vi "decode_request_from_serialport.vi"(6 "fast output index in":i32, 7 "fast output data in":dbl[][](array[numeric]), 8 "error in":errorcluster, 9 "FPGA VI Reference":refnum<k20>, 10 "request string":string, 11 "port name in":refnum<visa-resource-name>) -> (0 "error out":errorcluster, 2 "REQUEST_ID":u64, 3 "FPGA settings":T1={"Output settings"={"Relay Switch Matrix"=0, "Set output"=[0.0, 0.0, 0.0, 0.0], "set output?"=FALSE, "set relay matrix?"=FALSE}, "PID settings"={"PID input channel"=enum."PID Disabled", "PID output channel"=enum."PID Disabled", "PID gains"={"proportional gain"=0.0, "integral gain"=0.0, "derivative gain"=0.0, "filter coefficient"=0.0}, "PID output ranges"={"output high (Inf)"=0.0, "output low (-Inf)"=0.0}, "Setpoint for PID input chn"=0.0, "config PID gain?"=FALSE, "reset PID?"=FALSE, "config PID range?"=FALSE, "config PID input?"=FALSE, "config PID output?"=FALSE, "config PID setpoint?"=FALSE, "PID input scale factor"=1.0, "PID input offset"=0.0}, "NI9219 Settings"={"9219 Conversion Time"=enum."High Speed", "Input voltage range"=[0, 0, 0, 0], "config 9219 conversion time?"=FALSE, "config 9219 input range?"=FALSE}, "REQUEST_ID"=0, "requests"={"request_data"=FALSE, "request_system_status"=FALSE, "request_error_log"=FALSE}} {"REQUEST_ID" format="%x"; "NI9219 Settings"."Input voltage range" items=["+/- 60V", "+/- 15V", "+/- 4V", "+/- 1V", "+/- 125mV"]}, 4 "fast output index out":i32, 5 "fast output data out":dbl[][](array[numeric]))   [LabVIEW 2018]
uses:
  Type Def Ctrls/RT ctrls/FPGA parameter cluster.ctl
  Type Def Ctrls/FPGA ctrls/NI9219VoltageRange.ctl
  Type Def Ctrls/keywords for serial communication.ctl
  <vilib>/Utility/miscctls.llb/LVDateTimeRec.ctl
  <vilib>/FPGAPlugInAG/Dynamic/niLvFpga_Abort_Dynamic.vi
  <vilib>/FPGAPlugInAG/Dynamic/niLvFpga_Reset_Dynamic.vi
  <vilib>/FPGAPlugInAG/cRIO-9074/niLvFpga_Open_cRIO-9074.vi
  <vilib>/rvi/interface/common/dynamic/niFpgaDynamicAddResources.vi
  <vilib>/Utility/error.llb/Error Cluster From Error Code.vi
  <vilib>/rvi/errors/niLvFpgaAdjustHostInterfaceError.vi
  <vilib>/FPGAPlugInAG/Dynamic/niLvFpga_Close_Dynamic.vi
  <vilib>/nisyscfg/Close (System).vi
  <vilib>/rvi/interface/nirviMethod/nirviMethod.xnode
  <vilib>/rvi/interface/nirviOpenFPGA/nirviOpenFPGA.xnode
  FPGA Bitfiles/remotecontroller_FPGATarget_FPGAMain_RhGo+c1SRDI.lvbitx
  FPGA Main.vi
  <vilib>/rvi/interface/nirviReadWriteControl/nirviReadWriteControl.xnode
  <vilib>/rvi/interface/nirviCloseFPGA/nirviCloseFPGA.xnode
  <vilib>/nisyscfg/nisyscfg.lvlib
  NiFpgaLv.dll
  <vilib>/rvi/interface/Simulation/niFpgaSimulationCallBeginRW.vi
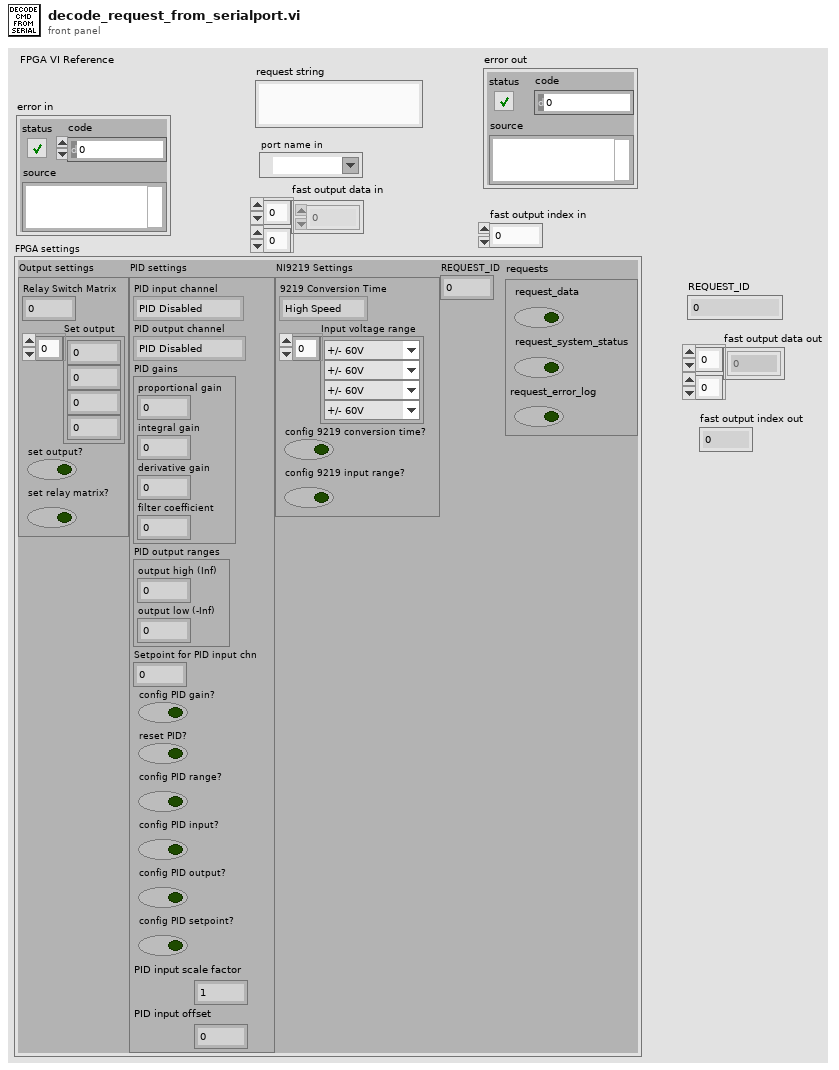
[diagram p1: front panel]
types:
  T1 = typedef "FPGA parameter cluster.ctl" = cluster{"Output settings":cluster{"Relay Switch Matrix":u32, "Set output":sgl[], "set output?":bool, "set relay matrix?":bool}, "PID settings":cluster{"PID input channel":enum16{"Output Channel 0", "Output Channel 1", "Output Channel 2", "Output Channel 3", "PID Disabled"}, "PID output channel":enum16{"Output Channel 0", "Output Channel 1", "Output Channel 2", "Output Channel 3", "PID Disabled"}, "PID gains":cluster{"proportional gain":sgl, "integral gain":sgl, "derivative gain":sgl, "filter coefficient":sgl}, "PID output ranges":cluster{"output high (Inf)":sgl, "output low (-Inf)":sgl}, "Setpoint for PID input chn":sgl, "config PID gain?":bool, "reset PID?":bool, "config PID range?":bool, "config PID input?":bool, "config PID output?":bool, "config PID setpoint?":bool, "PID input scale factor":sgl, "PID input offset":sgl}, "NI9219 Settings":cluster{"9219 Conversion Time":enum8{"High Speed", "Best 60 Hz Rejection", "Best 50 Hz Rejection", "High Resolution"}, "Input voltage range":T2[], "config 9219 conversion time?":bool, "config 9219 input range?":bool}, "REQUEST_ID":u64, "requests":cluster{"request_data":bool, "request_system_status":bool, "request_error_log":bool}}
  T2 = typedef "NI9219VoltageRange.ctl" = u8
  T3 = typedef "keywords for serial communication.ctl" = string[]
  T4 = enum16{"Safe State", "I/O with PID Control", "Fast Output Only", "NOT_READY"}
  T5 = typedef "LVDateTimeRec.ctl" = cluster{"fractional second":dbl, "second":i32, "minute":i32, "hour":i32, "day of month":i32, "month":i32, "year":i32, "day of week":i32, "day of year":i32, "DST":i32}
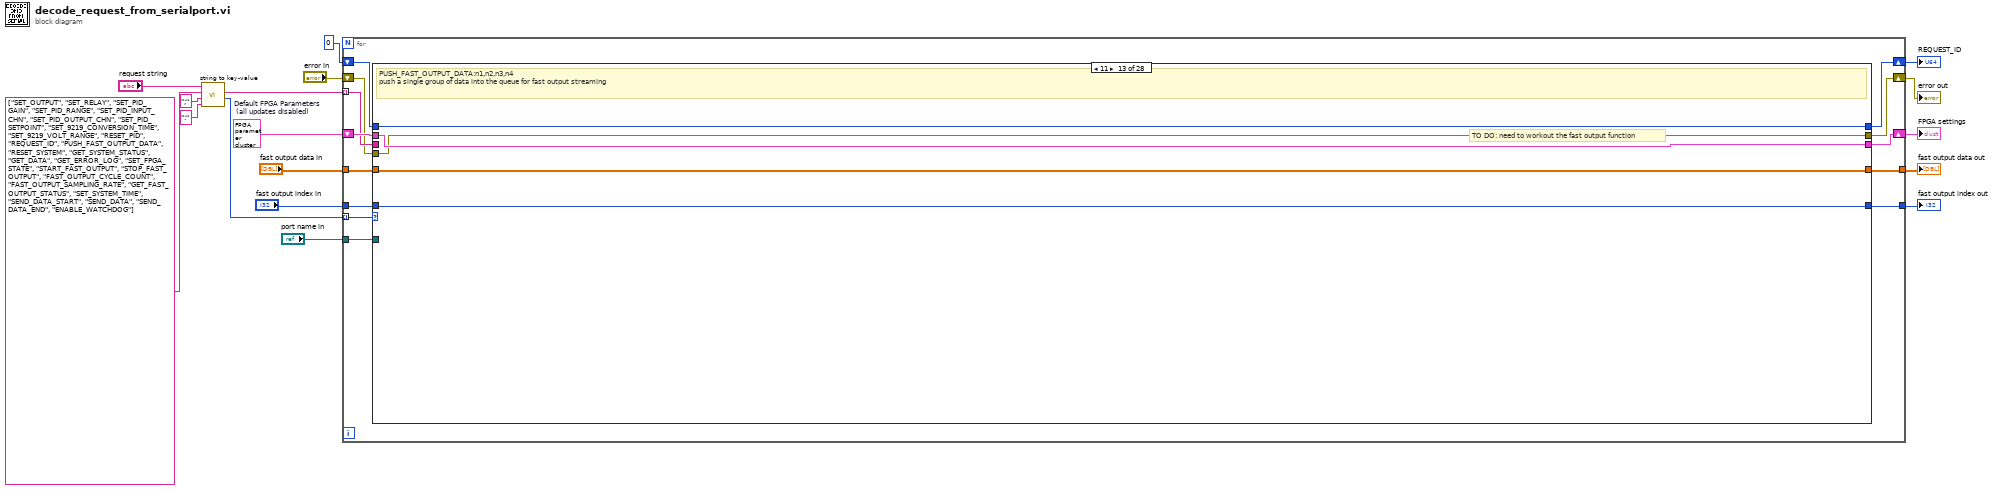
[diagram p0: block diagram]
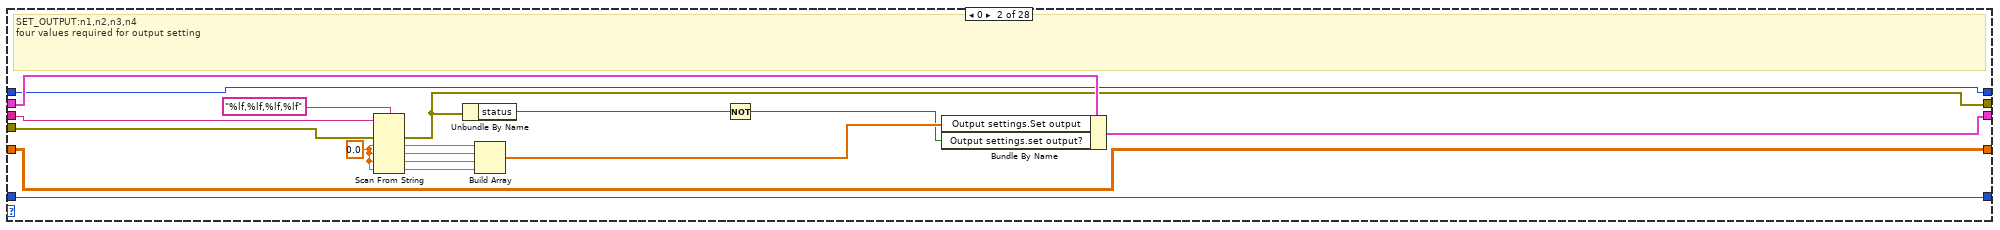
[diagram p3: hidden frame]
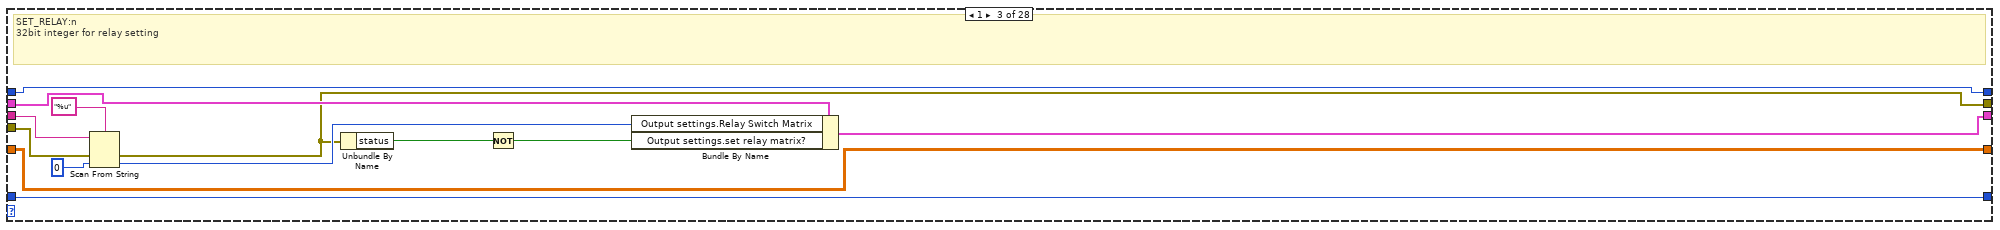
[diagram p4: hidden frame]
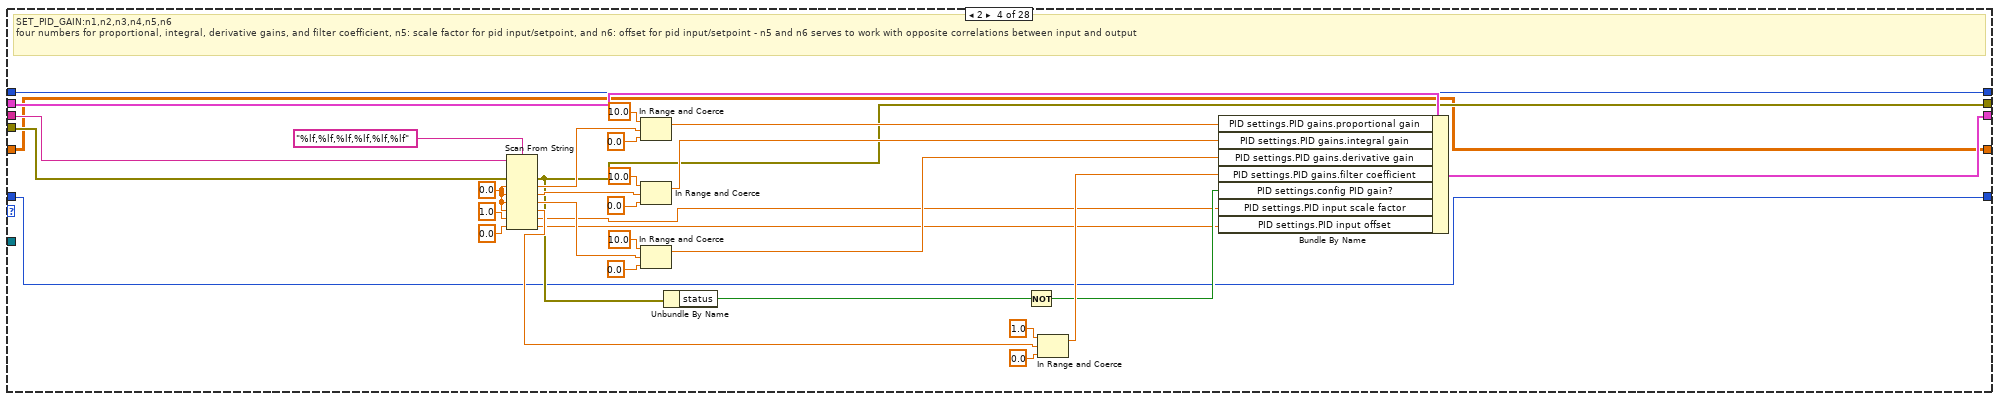
[diagram p5: hidden frame]
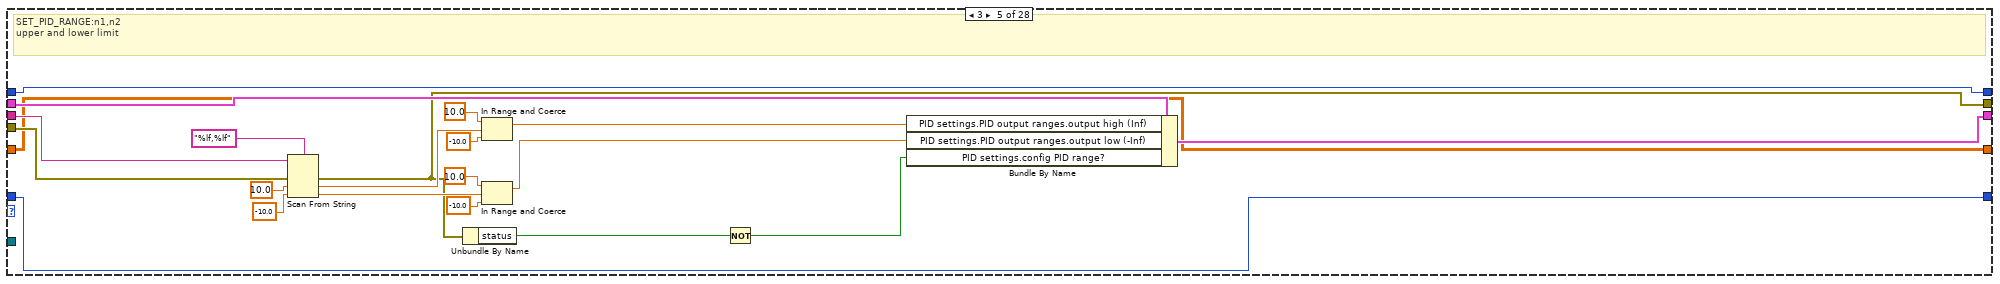
[diagram p6: hidden frame]
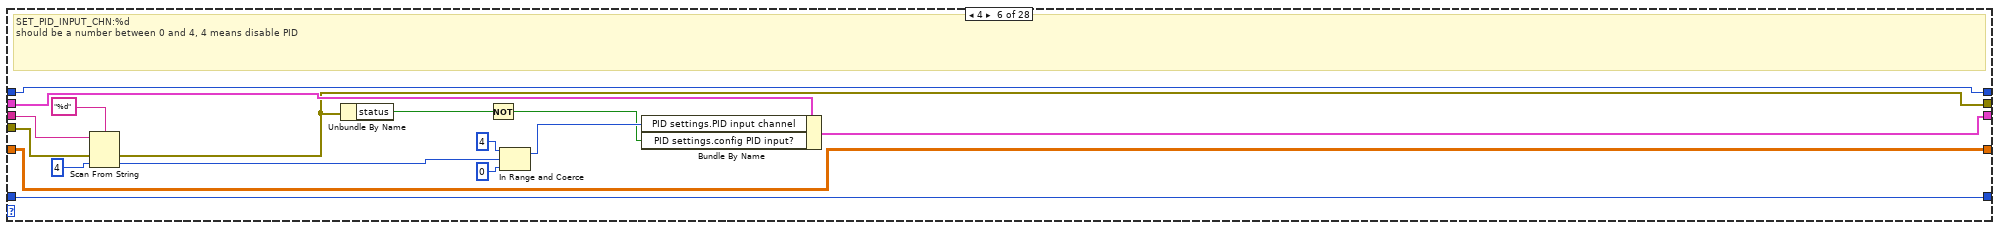
[diagram p7: hidden frame]
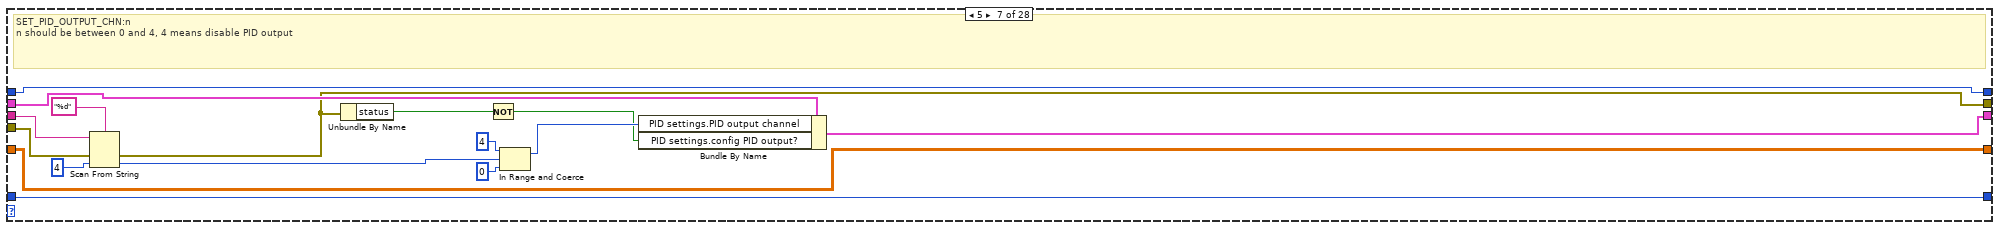
[diagram p8: hidden frame]
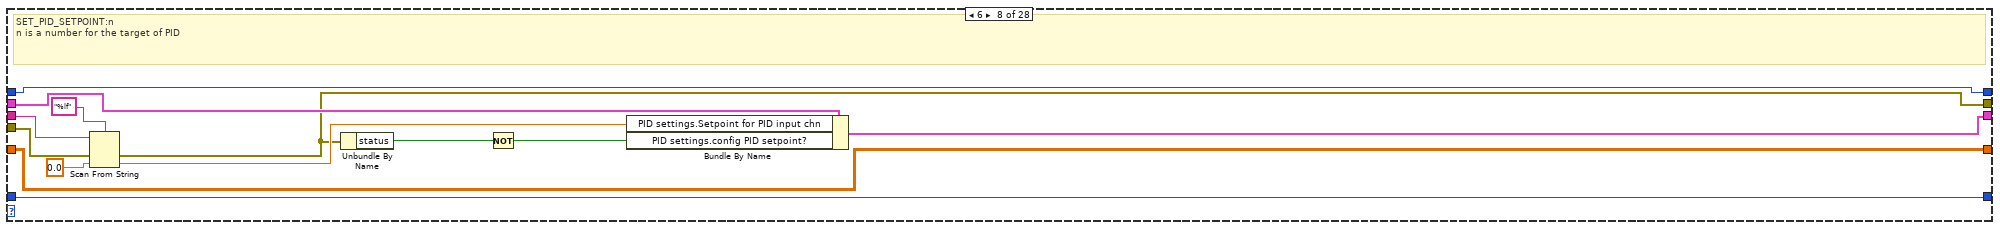
[diagram p9: hidden frame]
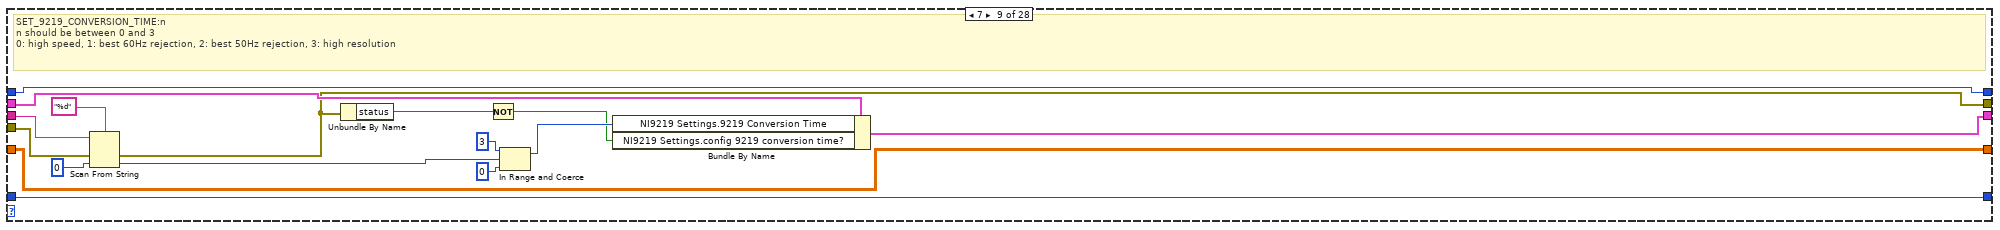
[diagram p10: hidden frame]
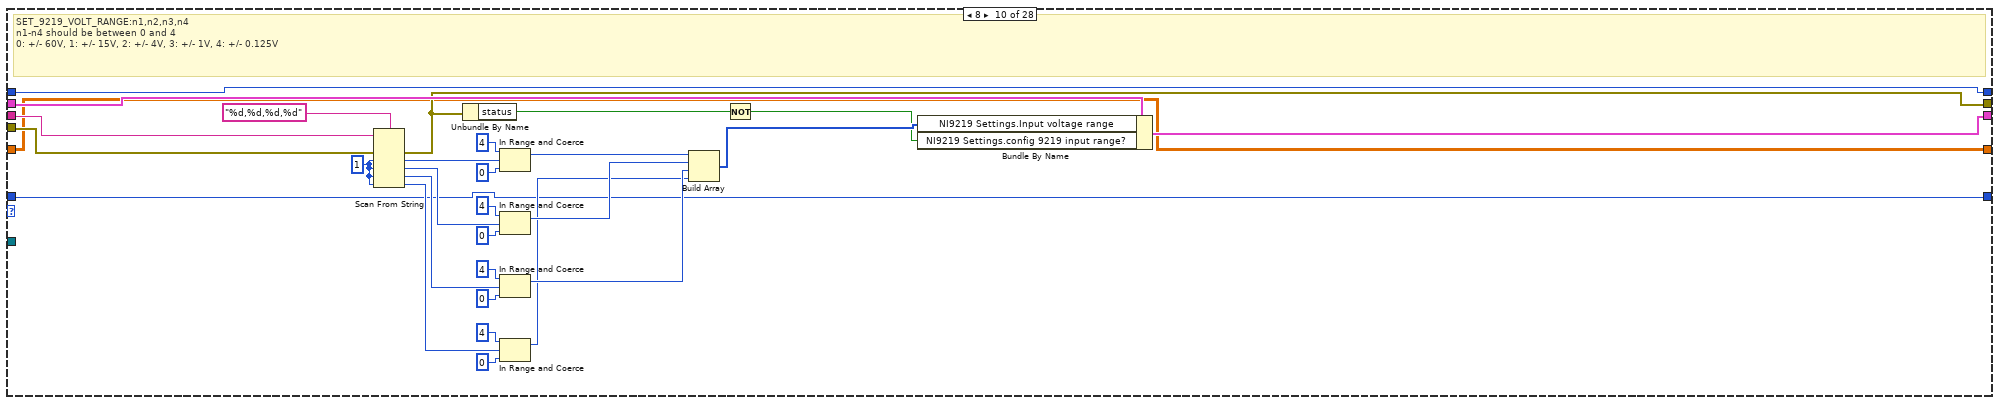
[diagram p11: hidden frame]
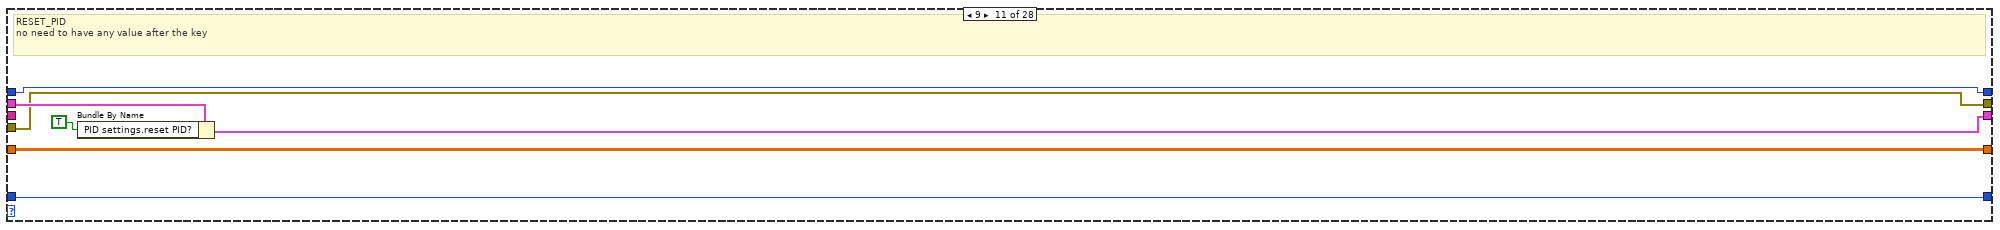
[diagram p12: hidden frame]
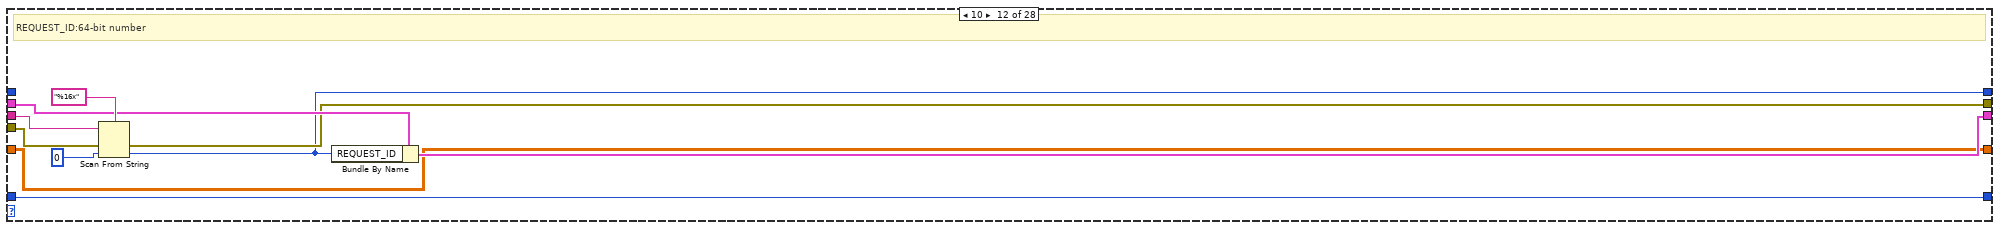
[diagram p13: hidden frame]
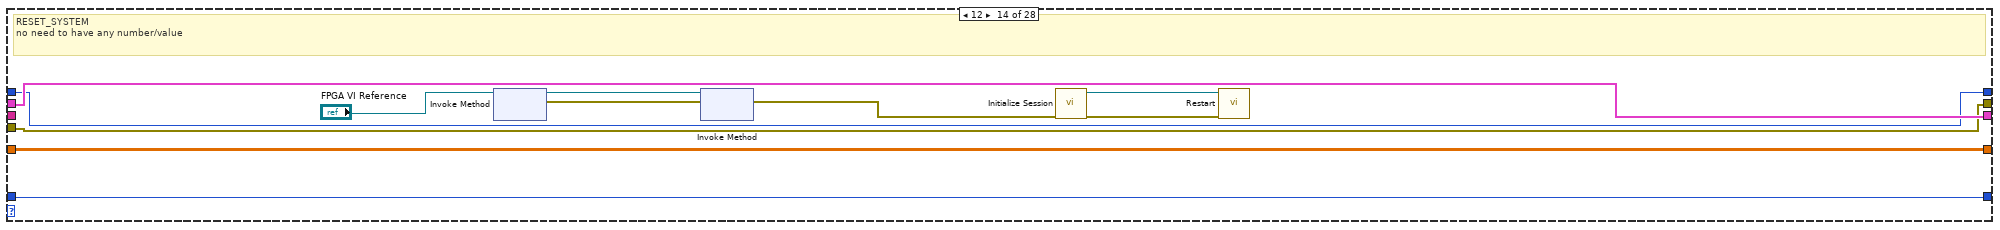
[diagram p14: hidden frame]
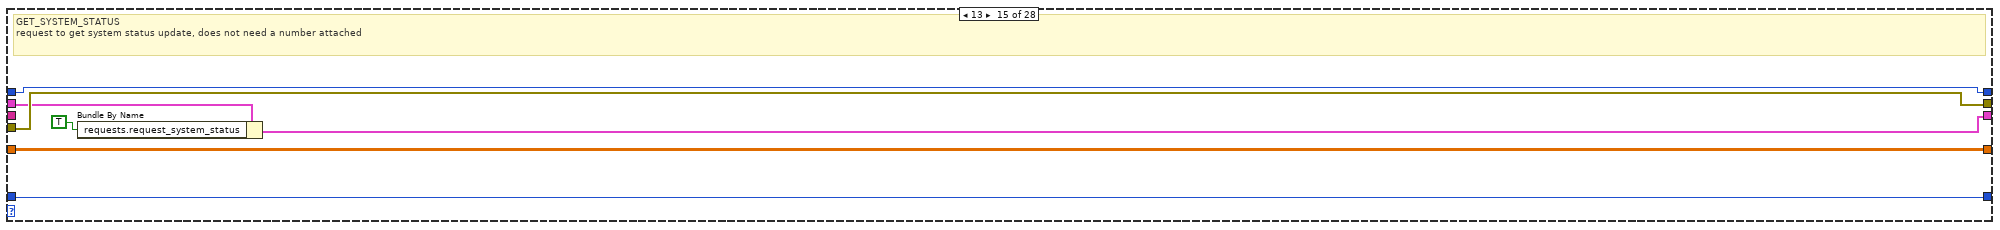
[diagram p15: hidden frame]
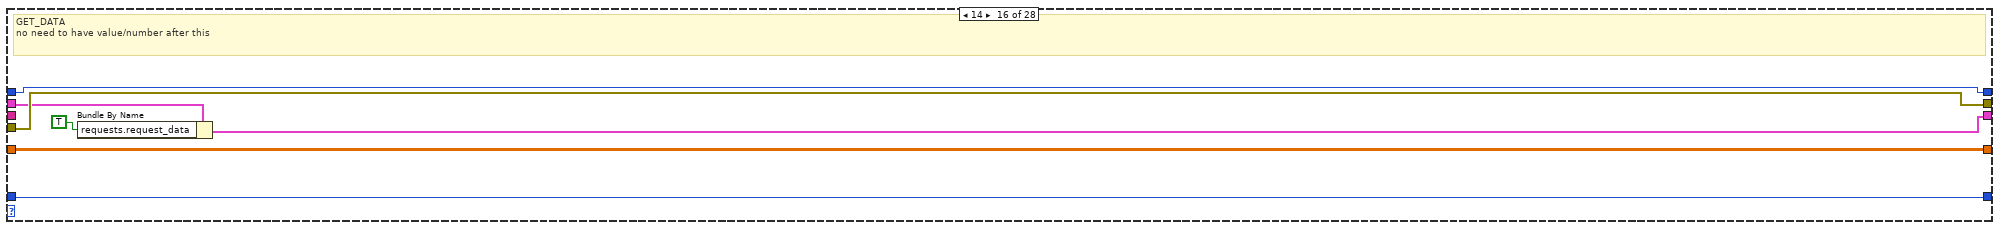
[diagram p16: hidden frame]
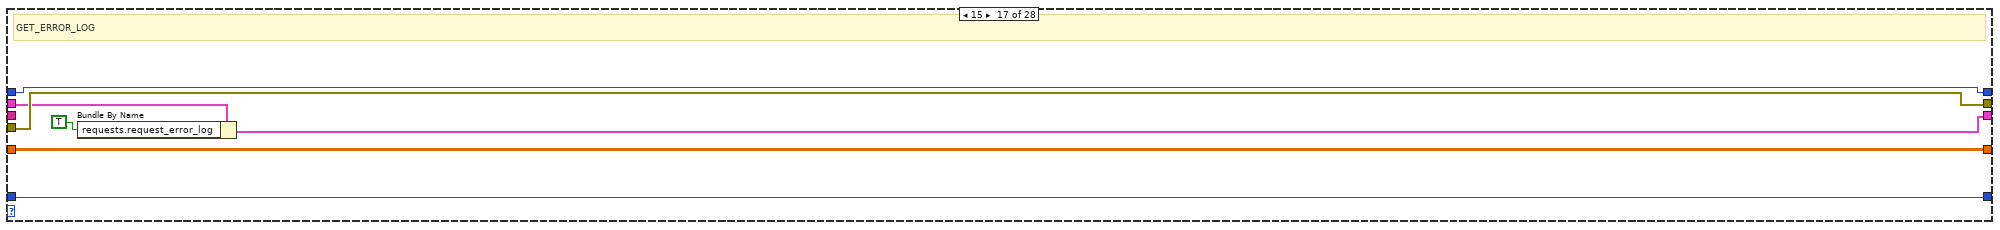
[diagram p17: hidden frame]
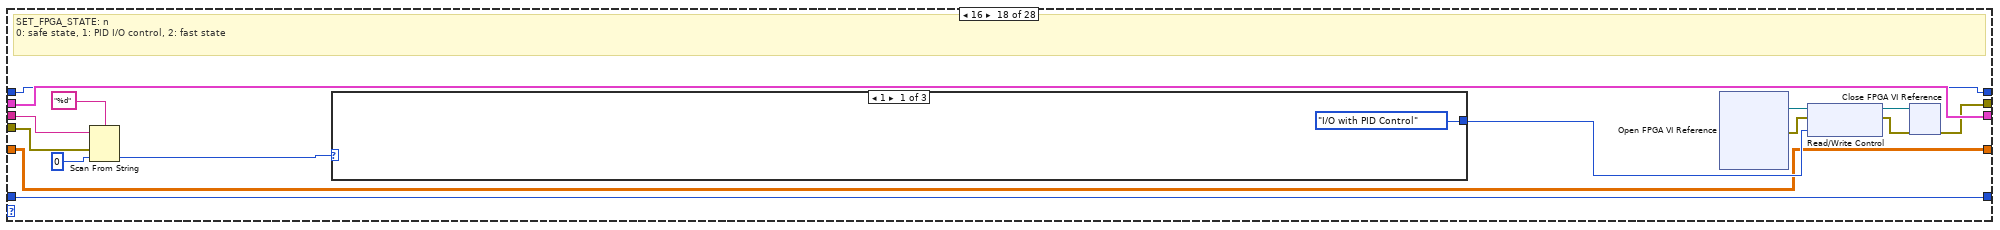
[diagram p18: hidden frame]
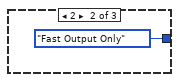
[diagram p19: hidden frame]
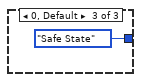
[diagram p20: hidden frame]
diagram:
  w15 = T1 {"Output settings"={"Relay Switch Matrix"=0, "Set output"=[0.0, 0.0, 0.0, 0.0], "set output?"=FALSE, "set relay matrix?"=FALSE}, "PID settings"={"PID input channel"=enum."PID Disabled", "PID output channel"=enum."PID Disabled", "PID gains"={"proportional gain"=0.0, "integral gain"=0.0, "derivative gain"=0.0, "filter coefficient"=0.0}, "PID output ranges"={"output high (Inf)"=0.0, "output low (-Inf)"=0.0}, "Setpoint for PID input chn"=0.0, "config PID gain?"=FALSE, "reset PID?"=FALSE, "config PID range?"=FALSE, "config PID input?"=FALSE, "config PID output?"=FALSE, "config PID setpoint?"=FALSE, "PID input scale factor"=1.0, "PID input offset"=0.0}, "NI9219 Settings"={"9219 Conversion Time"=enum."High Speed", "Input voltage range"=[1, 1, 1, 4], "config 9219 conversion time?"=FALSE, "config 9219 input range?"=FALSE}, "REQUEST_ID"=0, "requests"={"request_data"=FALSE, "request_system_status"=FALSE, "request_error_log"=FALSE}}  # Default FPGA Parameters  (all updates disabled)
  n1 = call "string to key-value.vi"("separation between key and value"=":", "separation between K-V sections"=";", "known key list"=T3 ["SET_OUTPUT", "SET_RELAY", "SET_PID_GAIN", "SET_PID_RANGE", "SET_PID_INPUT_CHN", "SET_PID_OUTPUT_CHN", "SET_PID_SETPOINT", "SET_9219_CONVERSION_TIME", "SET_9219_VOLT_RANGE", "RESET_PID", "REQUEST_ID", "PUSH_FAST_OUTPUT_DATA", "RESET_SYSTEM", "GET_SYSTEM_STATUS", "GET_DATA", "GET_ERROR_LOG", "SET_FPGA_STATE", "START_FAST_OUTPUT", "STOP_FAST_OUTPUT", "FAST_OUTPUT_CYCLE_COUNT", "FAST_OUTPUT_SAMPLING_RATE", "GET_FAST_OUTPUT_STATUS", "SET_SYSTEM_TIME", "SEND_DATA_START", "SEND_DATA", "SEND_DATA_END", "ENABLE_WATCHDOG"] ("key groups"), "input string"="request string") -> ("key index list"=w11:i32[], "value list"=w10:string[])  [unwired: 1 in, 1 out]
  n2 = for {
    shift-right: [w29] -> w16
    shift-left: w15 -> [w30]
    tunnel: w11 -> [w28] mode=indexing
    tunnel: w10 -> [w27] mode=indexing
    shift-right: [w25] -> w17
    shift-left: "error in" -> [w26]
    tunnel: "port name in" -> [w24]
    tunnel: [w23] -> w4
    tunnel: "fast output data in" -> [w22]
    tunnel: "fast output index in" -> [w21]
    tunnel: [w20] -> w3
    shift-right: [w19] -> w1
    shift-left: u64 0 ("default value 1") -> [w18]
    n3 = case shown="11" w28 {
      tunnel: w30 -> [w35 w52 w65 w97 w108 w128 w147 w160 w173 w193 w215 w222 w230 w241 w247 w254 w261 w269 w285 w290 w295 w300 w305 w311 w358 w370 w407 w414]
      tunnel: [w35 w51 w64 w77 w105 w126 w142 w158 w171 w187 w214 w221 w230 w241 w245 w253 w260 w269 w285 w290 w295 w300 w305 w311 w358 w370 w407 w414] -> w29
      tunnel: w27 -> [_ w50 w63 w96 w118 w134 w150 w163 w179 w208 _ w225 _ _ _ _ _ w273 _ _ _ _ _ w345 w356 w360 _ w418]
      tunnel: w26 -> [w34 w42 w58 w75 w104 w124 w141 w157 w170 w185 w212 w220 w229 w240 w248 w255 w262 w272 w284 w289 w294 w299 w304 w310 w355 w369 w406 w417]
      tunnel: [w34 w39 w56 w73 w102 w122 w138 w154 w167 w183 w212 w219 w229 w240 w248 w255 w262 w264 w284 w289 w294 w299 w304 w309 w354 w369 w406 w413] -> w25
      tunnel: w24 -> [_ _ _ _ _ _ _ _ _ _ _ _ _ _ _ _ _ _ _ _ _ _ _ _ _ _ _ _]
      tunnel: [w33 w38 w55 w72 w100 w121 w137 w153 w166 w182 w211 w218 w228 w233 w244 w251 w258 w268 w283 w288 w293 w298 w303 w308 w350 w367 w405 w412] -> w23
      tunnel: w22 -> [w33 w38 w55 w72 w100 w121 w137 w153 w166 w182 w211 w218 w228 w233 w244 w251 w258 w268 w283 w288 w293 w298 w303 w308 _ w366 w405 w412]
      tunnel: w21 -> [w32 w37 w54 w71 w99 w120 w136 w152 w165 w181 w210 w217 w227 w232 w243 w250 w257 w267 w282 w287 w292 w297 w302 w307 _ w365 _ w411]
      tunnel: [w32 w37 w54 w71 w99 w120 w136 w152 w165 w181 w210 w217 w227 w232 w243 w250 w257 w267 w282 w287 w292 w297 w302 w307 w349 w368 w402 w411] -> w20
      tunnel: [w31 w36 w53 w66 w98 w119 w135 w151 w164 w180 w209 w216 w226 w231 w242 w249 w256 w263 w281 w286 w291 w296 w301 w306 w346 w359 w401 w408] -> w19
      tunnel: w18 -> [w31 w36 w53 w66 w98 w119 w135 w151 w164 w180 w209 _ w226 w231 w242 w249 w256 w263 w281 w286 w291 w296 w301 w306 w346 w359 w401 w408]
      frame -1, Default {
      }
      frame 0 {
        w48 = 0.0 ("default value 1")
        # "SET_OUTPUT:n1,n2,n3,n4\nfour values required for output setting"
        n4 = Scan From String(format string="%lf,%lf,%lf,%lf", input string=w50, error in=w42, default 1=w48, default 2=w48, default 3=w48, default 4=w48) -> (error out=w39:errorcluster, output 1=w47:dbl, output 2=w46:dbl, output 3=w45:dbl, output 4=w44:dbl)  [unwired: 1 in, 2 out]
        n5 = Unbundle By Name(w39) -> ("status"=w41:bool)
        n6 = Build Array(w47, w46, w45, w44) -> (w43:dbl[])
        n7 = Not(x=w41) -> (.not. x?=w40:bool)
        n8 = Bundle By Name(cluster=w52, "Output settings.Set output"=w43, "Output settings.set output?"=w40) -> (w51:T1)
      }
      frame 1 {
        # "SET_RELAY:n\n32bit integer for relay setting"
        n9 = Scan From String(format string="%u", input string=w63, error in=w58, default 1=u32 0 ("default value 1")) -> (error out=w56:errorcluster, output 1=w60:u32)  [unwired: 1 in, 2 out]
        n10 = Unbundle By Name(w56) -> ("status"=w59:bool)
        n11 = Not(x=w59) -> (.not. x?=w57:bool)
        n12 = Bundle By Name(cluster=w65, "Output settings.Relay Switch Matrix"=w60, "Output settings.set relay matrix?"=w57) -> (w64:T1)
      }
      frame 2 {
        w94 = 0.0 ("default value 4")
        # "SET_PID_GAIN:n1,n2,n3,n4,n5,n6\nfour numbers for proportional, integral, derivative gains, and filter coefficient, n5: scale factor for pid input/setpoint, and n6: offset for pid input/setpoint - n5 and n6 serves to work with opposite correlations between input and output"
        n13 = Scan From String(format string="%lf,%lf,%lf,%lf,%lf,%lf", input string=w96, error in=w75, default 1=w94, default 2=w94, default 3=w94, default 4=w94, default 5=1.0 ("default value 5"), default 6=0.0 ("default value 6")) -> (error out=w73:errorcluster, output 1=w93:dbl, output 2=w83:dbl, output 3=w81:dbl, output 4=w78:dbl, output 5=w68:dbl, output 6=w67:dbl)  [unwired: 1 in, 2 out]
        n14 = In Range and Coerce(upper limit=10.0, x=w93, lower limit=0.0) -> (coerced(x)=w90:dbl)  [unwired: 1 out]
        n15 = In Range and Coerce(upper limit=10.0, x=w83, lower limit=0.0) -> (coerced(x)=w82:dbl)  [unwired: 1 out]
        n16 = In Range and Coerce(upper limit=10.0, x=w81, lower limit=0.0) -> (coerced(x)=w80:dbl)  [unwired: 1 out]
        n17 = Unbundle By Name(w73) -> ("status"=w76:bool)
        n18 = Not(x=w76) -> (.not. x?=w74:bool)
        n19 = In Range and Coerce(upper limit=1.0, x=w78, lower limit=0.0) -> (coerced(x)=w79:dbl)  [unwired: 1 out]
        n20 = Bundle By Name(cluster=w97, "PID settings.PID gains.proportional gain"=w90, "PID settings.PID gains.integral gain"=w82, "PID settings.PID gains.derivative gain"=w80, "PID settings.PID gains.filter coefficient"=w79, "PID settings.config PID gain?"=w74, "PID settings.PID input scale factor"=w68, "PID settings.PID input offset"=w67) -> (w77:T1)
      }
      frame 3 {
        # "SET_PID_RANGE:n1,n2\nupper and lower limit"
        n21 = Scan From String(format string="%lf,%lf", input string=w118, error in=w104, default 1=10.0 ("default value 1"), default 2=-10.0 ("default value 2")) -> (error out=w102:errorcluster, output 1=w114:dbl, output 2=w109:dbl)  [unwired: 1 in, 2 out]
        n22 = Unbundle By Name(w102) -> ("status"=w103:bool)
        n23 = In Range and Coerce(upper limit=10.0, x=w114, lower limit=-10.0) -> (coerced(x)=w107:dbl)  [unwired: 1 out]
        n24 = In Range and Coerce(upper limit=10.0, x=w109, lower limit=-10.0) -> (coerced(x)=w106:dbl)  [unwired: 1 out]
        n25 = Not(x=w103) -> (.not. x?=w101:bool)
        n26 = Bundle By Name(cluster=w108, "PID settings.PID output ranges.output high (Inf)"=w107, "PID settings.PID output ranges.output low (-Inf)"=w106, "PID settings.config PID range?"=w101) -> (w105:T1)
      }
      frame 4 {
        # "SET_PID_INPUT_CHN:%d\nshould be a number between 0 and 4, 4 means disable PID"
        n27 = Scan From String(format string="%d", input string=w134, error in=w124, default 1=4 ("default value 1")) -> (error out=w122:errorcluster, output 1=w131:i32)  [unwired: 1 in, 2 out]
        n28 = Unbundle By Name(w122) -> ("status"=w125:bool)
        n29 = Not(x=w125) -> (.not. x?=w123:bool)
        n30 = In Range and Coerce(upper limit=4, x=w131, lower limit=0) -> (coerced(x)=w127:i32)  [unwired: 1 out]
        n31 = Bundle By Name(cluster=w128, "PID settings.PID input channel"=w127, "PID settings.config PID input?"=w123) -> (w126:T1)
      }
      frame 5 {
        # "SET_PID_OUTPUT_CHN:n\nn should be between 0 and 4, 4 means disable PID output"
        n32 = Scan From String(format string="%d", input string=w150, error in=w141, default 1=4 ("default value 1")) -> (error out=w138:errorcluster, output 1=w146:i32)  [unwired: 1 in, 2 out]
        n33 = Unbundle By Name(w138) -> ("status"=w140:bool)
        n34 = Not(x=w140) -> (.not. x?=w139:bool)
        n35 = In Range and Coerce(upper limit=4, x=w146, lower limit=0) -> (coerced(x)=w143:i32)  [unwired: 1 out]
        n36 = Bundle By Name(cluster=w147, "PID settings.PID output channel"=w143, "PID settings.config PID output?"=w139) -> (w142:T1)
      }
      frame 6 {
        # "SET_PID_SETPOINT:n\nn is a number for the target of PID"
        n37 = Scan From String(format string="%lf", input string=w163, error in=w157, default 1=0.0 ("default value 1")) -> (error out=w154:errorcluster, output 1=w159:dbl)  [unwired: 1 in, 2 out]
        n38 = Unbundle By Name(w154) -> ("status"=w156:bool)
        n39 = Not(x=w156) -> (.not. x?=w155:bool)
        n40 = Bundle By Name(cluster=w160, "PID settings.Setpoint for PID input chn"=w159, "PID settings.config PID setpoint?"=w155) -> (w158:T1)
      }
      frame 7 {
        # "SET_9219_CONVERSION_TIME:n\nn should be between 0 and 3\n0: high speed, 1: best 60Hz rejection, 2: best 50Hz rejection, 3: high resolution"
        n41 = Scan From String(format string="%d", input string=w179, error in=w170, default 1=0 ("default value 1")) -> (error out=w167:errorcluster, output 1=w176:i32)  [unwired: 1 in, 2 out]
        n42 = Unbundle By Name(w167) -> ("status"=w169:bool)
        n43 = Not(x=w169) -> (.not. x?=w168:bool)
        n44 = In Range and Coerce(upper limit=3, x=w176, lower limit=0) -> (coerced(x)=w172:i32)  [unwired: 1 out]
        n45 = Bundle By Name(cluster=w173, "NI9219 Settings.9219 Conversion Time"=w172, "NI9219 Settings.config 9219 conversion time?"=w168) -> (w171:T1)
      }
      frame 8 {
        w206 = 1 ("default value 1")
        # "SET_9219_VOLT_RANGE:n1,n2,n3,n4\nn1-n4 should be between 0 and 4\n0: +/- 60V, 1: +/- 15V, 2: +/- 4V, 3: +/- 1V, 4: +/- 0.125V"
        n46 = Scan From String(format string="%d,%d,%d,%d", input string=w208, error in=w185, default 1=w206, default 2=w206, default 3=w206, default 4=w206) -> (error out=w183:errorcluster, output 1=w205:i32, output 2=w195:i32, output 3=w196:i32, output 4=w194:i32)  [unwired: 1 in, 2 out]
        n47 = Unbundle By Name(w183) -> ("status"=w186:bool)
        n48 = In Range and Coerce(upper limit=4, x=w205, lower limit=0) -> (coerced(x)=w192:i32)  [unwired: 1 out]
        n49 = In Range and Coerce(upper limit=4, x=w195, lower limit=0) -> (coerced(x)=w191:i32)  [unwired: 1 out]
        n50 = In Range and Coerce(upper limit=4, x=w196, lower limit=0) -> (coerced(x)=w190:i32)  [unwired: 1 out]
        n51 = In Range and Coerce(upper limit=4, x=w194, lower limit=0) -> (coerced(x)=w189:i32)  [unwired: 1 out]
        n52 = Build Array(w192, w191, w190, w189) -> (w188:i32[])
        n53 = Not(x=w186) -> (.not. x?=w184:bool)
        n54 = Bundle By Name(cluster=w193, "NI9219 Settings.Input voltage range"=w188, "NI9219 Settings.config 9219 input range?"=w184) -> (w187:T1)
      }
      frame 9 {
        # "RESET_PID\nno need to have any value after the key"
        n55 = Bundle By Name(cluster=w215, "PID settings.reset PID?"=TRUE) -> (w214:T1)
      }
      frame 10 {
        # "REQUEST_ID:64-bit number"
        n56 = Scan From String(format string="%16x", input string=w225, error in=w220, default 1=u64 0 ("default value 1")) -> (error out=w219:errorcluster, output 1=w216:u64)  [unwired: 1 in, 2 out]
        n57 = Bundle By Name(cluster=w222, "REQUEST_ID"=w216) -> (w221:T1)
      }
      frame 11 {
        # "TO DO: need to workout the fast output function"
        # "PUSH_FAST_OUTPUT_DATA:n1,n2,n3,n4\npush a single group of data into the queue for fast output streaming"
      }
      frame 12 {
        # "RESET_SYSTEM\nno need to have any number/value"
        n58 = xnode "Invoke Method"("FPGA VI Reference In"="FPGA VI Reference") -> ("FPGA VI Reference Out"=w235:refnum<k20>, "error out"=w236:errorcluster)  [unwired: 1 in]
        n59 = xnode "Invoke Method"("FPGA VI Reference In"=w235, "error in"=w236) -> ("error out"=w234:errorcluster)  [unwired: 1 out]
        n60 = call <vilib>:"Initialize Session.vi"("error in (no error)"=w234) -> ("error out"=w238:errorcluster, "Session out"=w239:refnum<k21>)  [unwired: 9 in]
        n61 = call <vilib>:"Restart.vi"("error in (no error)"=w238, "Session in"=w239) -> ()  [unwired: 7 in, 3 out]
      }
      frame 13 {
        # "GET_SYSTEM_STATUS\nrequest to get system status update, does not need a number attached"
        n62 = Bundle By Name(cluster=w247, "requests.request_system_status"=TRUE) -> (w245:T1)
      }
      frame 14 {
        # "GET_DATA\nno need to have value/number after this"
        n63 = Bundle By Name(cluster=w254, "requests.request_data"=TRUE) -> (w253:T1)
      }
      frame 15 {
        # "GET_ERROR_LOG"
        n64 = Bundle By Name(cluster=w261, "requests.request_error_log"=TRUE) -> (w260:T1)
      }
      frame 16 {
        # "SET_FPGA_STATE: n\n0: safe state, 1: PID I/O control, 2: fast state"
        n65 = Scan From String(format string="%d", input string=w273, error in=w272, default 1=0 ("default value 1")) -> (output 1=w271:i32)  [unwired: 1 in, 3 out]
        n66 = case shown="1" w271 {
          tunnel: [T4."I/O with PID Control" ("FPGA state") T4."Fast Output Only" ("FPGA state") T4."Safe State" ("FPGA state")] -> w270
          frame 1 {
          }
          frame 2 {
          }
          frame 0, Default {
          }
        }
        n67 = xnode "Open FPGA VI Reference"() -> ("FPGA VI Reference Out"=w277:refnum<k20>, "error out"=w276:errorcluster)  [unwired: 2 in]
        n68 = xnode "Read/Write Control"("FPGA VI Reference In"=w277, "error in"=w276, "FPGA state"=w270) -> ("FPGA VI Reference Out"=w266:refnum<k20>, "error out"=w265:errorcluster)
        n69 = xnode "Close FPGA VI Reference"("FPGA VI Reference In"=w266, "error in"=w265) -> ("error out"=w264:errorcluster)
      }
      frame 17 {
      }
      frame 18 {
      }
      frame 19 {
      }
      frame 20 {
      }
      frame 21 {
      }
      frame 22 {
        w343 = 0 ("default value 2")
        # "SET_SYSTEM_TIME:n1/n2/n3/n4/n5/n6\nn1: Month, n2: Day, n3: Year, n4: hour, n5: minute, n6: second, 24 hour format"
        n70 = Scan From String(format string="%d/%d/%d/%d/%d/%d", input string=w345, default 1=w343, default 2=w343, default 3=w343, default 4=w343, default 5=w343, default 6=w343) -> (output 1=w342:i32, output 2=w337:i32, output 3=w334:i32, output 4=w331:i32, output 5=w328:i32, output 6=w325:i32)  [unwired: 2 in, 3 out]
        n71 = In Range and Coerce(upper limit=12, x=w342, lower limit=1) -> (coerced(x)=w322:i32)  [unwired: 1 out]
        n72 = In Range and Coerce(upper limit=31, x=w337, lower limit=1) -> (coerced(x)=w320:i32)  [unwired: 1 out]
        n73 = In Range and Coerce(upper limit=23, x=w331, lower limit=0) -> (coerced(x)=w319:i32)  [unwired: 1 out]
        n74 = In Range and Coerce(upper limit=59, x=w328, lower limit=0) -> (coerced(x)=w318:i32)  [unwired: 1 out]
        n75 = In Range and Coerce(upper limit=59, x=w325, lower limit=0) -> (coerced(x)=w317:i32)  [unwired: 1 out]
        n76 = In Range and Coerce(upper limit=9999, x=w334, lower limit=0) -> (coerced(x)=w321:i32)  [unwired: 1 out]
        n77 = Bundle By Name(cluster=T5 {"fractional second"=0.0, "second"=0, "minute"=0, "hour"=0, "day of month"=0, "month"=0, "year"=0, "day of week"=0, "day of year"=0, "DST"=0} ("date time rec"), "year"=w321, "month"=w322, "day of month"=w320, "hour"=w319, "minute"=w318, "second"=w317) -> (w316:T5)
        n78 = Date/Time To Seconds(2:w316) -> (0:w324:timestamp)  [unwired: 1 in]
        n79 = call <vilib>:"Initialize Session.vi"("error in (no error)"=w310) -> ("error out"=w312:errorcluster, "Session out"=w315:refnum<k21>)  [unwired: 9 in]
        n80 = call <vilib>:"Set Time.vi"("error in (no error)"=w312, "Time"=w324, "Session in (localhost)"=w315) -> ("error out"=w314:errorcluster, "Session out"=w313:refnum<k21>)  [unwired: 5 in, 2 out]
        n81 = call-poly <vilib>:"Close.vi"("error in (no error)"=w314, "Session in"=w313) -> ("error out"=w309:errorcluster)  [unwired: 9 in]
      }
      frame 23 {
        w349 = 0 ("default value 1")
        # "SEND_DATA_START:n\nn is the total number of points"
        n82 = Scan From String(format string="%d", input string=w356, error in=w355, default 1=w349) -> (error out=w354:errorcluster, output 1=w352:i32)  [unwired: 1 in, 2 out]
        n83 = Greater Than 0?(x=w352) -> (x > 0?=w353:bool)
        n84 = Select(t=w352, s=w353, f=w349) -> (s? t:f=w347:i32)
        n85 = Initialize Array(0.0 ("element"), w347, 5 ("dimension size")) -> (w350:dbl[][])
      }
      frame 24 {
        # "SEND_DATA:n1,n2,n3,n4,n5\nn1,n2,n3,n4: voltage for output channels, n5: duration (counts of ticks, minimal 1)"
        n86 = Array Size(array=w366) -> (size(s)=w363:i32[])
        n87 = Index Array(array=w363, index=0) -> (element=w361:i32)
        n88 = Less?(x=w365, y=w361) -> (x < y?=w364:bool)
        n89 = case shown="True" w364 {
          tunnel: [w372 w398] -> w368
          tunnel: [w371 w397] -> w367
          tunnel: w366 -> [w371 w393]
          tunnel: w365 -> [w372 w381]
          tunnel: w360 -> [_ w373]
          frame False {
          }
          frame True {
            w392 = 1 ("default value 2")
            w374 = 0.0 ("default value 1")
            n90 = Increment(x=w381) -> (x+1=w398:i32)
            n91 = Scan From String(format string="%lf,%lf,%lf,%lf,%d", input string=w373, default 1=w374, default 2=w374, default 3=w374, default 4=w374, default 5=w392) -> (output 1=w396:dbl, output 2=w384:dbl, output 3=w383:dbl, output 4=w382:dbl, output 5=w385:i32)  [unwired: 2 in, 3 out]
            n92 = Greater Or Equal?(x=w385, y=w392) -> (x >= y?=w399:bool)
            n93 = In Range and Coerce(upper limit=10.0, x=w396, lower limit=-10.0) -> (coerced(x)=w380:dbl)  [unwired: 1 out]
            n94 = In Range and Coerce(upper limit=10.0, x=w384, lower limit=-10.0) -> (coerced(x)=w379:dbl)  [unwired: 1 out]
            n95 = In Range and Coerce(upper limit=10.0, x=w383, lower limit=-10.0) -> (coerced(x)=w378:dbl)  [unwired: 1 out]
            n96 = In Range and Coerce(upper limit=10.0, x=w382, lower limit=-10.0) -> (coerced(x)=w377:dbl)  [unwired: 1 out]
            n97 = Select(t=w385, s=w399, f=w392) -> (s? t:f=w376:i32)
            n98 = Build Array(w380, w379, w378, w377, w376) -> (w375:dbl[])
            n99 = Replace Array Subset(array=w393, new element=w375, index (row)=w381) -> (w397:dbl[][])  [unwired: 1 in]
          }
        }
      }
      frame 25 {
        # "SEND_DATA_END"
        n100 = Array Size(array=w405) -> (size(s)=w404:i32[])
        n101 = Index Array(array=w404, index=0) -> (element=w402:i32)
      }
      frame 26 {
        # "SWITCH_WATCHDOG"
        n102 = Scan From String(format string="%d", input string=w418, error in=w417, default 1=1 ("default value 1")) -> (error out=w413:errorcluster, output 1=w416:i32)  [unwired: 1 in, 2 out]
        n103 = xnode "Open FPGA VI Reference"() -> ("FPGA VI Reference Out"=w422:refnum<k20>, "error out"=w421:errorcluster)  [unwired: 2 in]
        n104 = Not Equal To 0?(x=w416) -> (x != 0?=w415:bool)
        n105 = xnode "Read/Write Control"("FPGA VI Reference In"=w422, "error in"=w421, "Enable Watchdog"=w415) -> ("FPGA VI Reference Out"=w410:refnum<k20>, "error out"=w409:errorcluster)
        n106 = xnode "Close FPGA VI Reference"("FPGA VI Reference In"=w410, "error in"=w409) -> ()  [unwired: 1 out]
      }
    }
  }
  "FPGA settings" <- w16
  "error out" <- w17
  "fast output data out" <- w4
  "fast output index out" <- w3
  "REQUEST_ID" <- w1
